vi "writeAimingBeamSetting.vi"(8 "error in":errorcluster, 11 "Aiming Beam Cluster":T1={"Aiming Beam COM Port"="COM3", "Min Current"=0.0, "Max Current"=63.0, "Default Current"=20.0, "Frequency(Hz)"=15}) -> (0 "error out":errorcluster)   [LabVIEW 2020]
uses:
  SubVI/TecLaserControl/AimingBeam.ctl
  <vilib>/Utility/config.llb/Write Key (String).vi
  <vilib>/Utility/config.llb/Write Key (Double).vi
  <vilib>/Utility/config.llb/Write Key (U32).vi
  <vilib>/Utility/config.llb/NI_LVConfig.lvlib
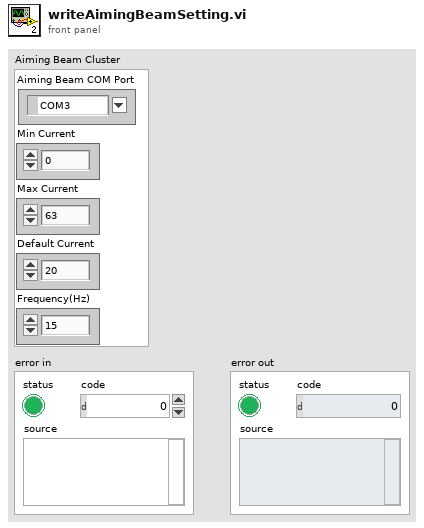
[diagram p1: front panel]
types:
  T1 = typedef "AimingBeam.ctl" = cluster{"Aiming Beam COM Port":refnum<visa-resource-name>, "Min Current":dbl, "Max Current":dbl, "Default Current":dbl, "Frequency(Hz)":u32}
  T2 = typedef "NI_LVConfig.lvlib/Config Data RefNum.ctl" = refnum<k1>
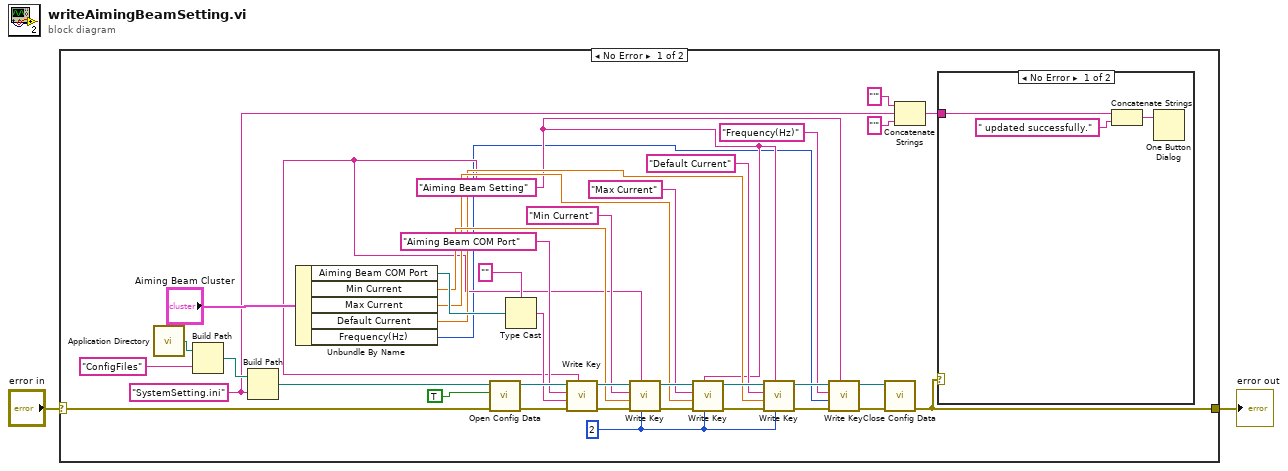
[diagram p0: block diagram]
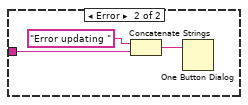
[diagram p2: hidden frame]
diagram:
  n1 = case shown="No Error" "error in" {
    selector: "error in" -> [w31 w47]
    tunnel: [w4 w47] -> w2
    frame No Error {
      w3 = i16 2 ("precision (6)")
      w8 = "Aiming Beam Setting" ("section")
      w28 = "SystemSetting.ini" ("name or relative path")
      n2 = call <vilib>:"Application Directory.vi"() -> ("Application Directory"=w34:path)
      n3 = Build Path(base path=w34, name or relative path="ConfigFiles") -> (appended path=w32:path)
      n4 = Build Path(base path=w32, name or relative path=w28) -> (appended path=w30:path)
      n5 = Unbundle By Name("Aiming Beam Cluster") -> ("Aiming Beam COM Port"=w39:refnum<visa-resource-name>, "Min Current"=w20:dbl, "Max Current"=w16:dbl, "Default Current"=w12:dbl, "Frequency(Hz)"=w7:u32)
      n6 = call <vilib>:"Open Config Data.vi"("error in (no error)"=w31, "create file if necessary (T)"=TRUE, "configuration file path"=w30) -> ("error out"=w27:errorcluster, "refnum"=w26:T2)  [unwired: 6 in, 1 out]
      n7 = Type Cast(type="", x=w39) -> (*(type *) &x=w24:string)
      n8 = call-poly <vilib>:"Write Key.vi"("section"=w8, "error in (no error)"=w27, "value"=w24, "key"="Aiming Beam COM Port", "refnum"=w26) -> ("error out"=w22:errorcluster, "refnum out"=w23:T2)  [unwired: 4 in, 1 out]
      n9 = call-poly <vilib>:"Write Key.vi"("precision (6)"=w3, "section"=w8, "error in (no error)"=w22, "value"=w20, "key"="Min Current", "refnum"=w23) -> ("error out"=w18:errorcluster, "refnum out"=w19:T2)  [unwired: 3 in, 1 out]
      n10 = call-poly <vilib>:"Write Key.vi"("precision (6)"=w3, "section"=w8, "error in (no error)"=w18, "value"=w16, "key"="Max Current", "refnum"=w19) -> ("error out"=w14:errorcluster, "refnum out"=w15:T2)  [unwired: 3 in, 1 out]
      n11 = call-poly <vilib>:"Write Key.vi"("precision (6)"=w3, "section"=w8, "error in (no error)"=w14, "value"=w12, "key"="Default Current", "refnum"=w15) -> ("error out"=w10:errorcluster, "refnum out"=w11:T2)  [unwired: 3 in, 1 out]
      n12 = call-poly <vilib>:"Write Key.vi"("section"=w8, "error in (no error)"=w10, "value"=w7, "key"="Frequency(Hz)", "refnum"=w11) -> ("error out"=w5:errorcluster, "refnum out"=w6:T2)  [unwired: 4 in, 1 out]
      n13 = call <vilib>:"Close Config Data.vi"("error in (no error)"=w5, "refnum"=w6) -> ("error out"=w4:errorcluster)  [unwired: 8 in, 1 out]
      n14 = Concatenate Strings("'" ("string"), w28, "'" ("string")) -> (w35:string)
      n15 = case shown="No Error" w4 {
        tunnel: w35 -> [w43 w45]
        frame No Error {
          n16 = Concatenate Strings(w43, " updated successfully." ("string")) -> (w41:string)
          n17 = One Button Dialog(message=w41) -> ()  [unwired: 1 in, 1 out]
        }
        frame Error {
          n18 = Concatenate Strings("Error updating " ("string"), w45) -> (w46:string)
          n19 = One Button Dialog(message=w46) -> ()  [unwired: 1 in, 1 out]
        }
      }
    }
    frame Error {
    }
  }
  "error out" <- w2
